vi "Arreglos.vi"() -> ()   [LabVIEW 2020]
uses:
  868cc0ce-591d-4479-aae9-2e439e702293.vi
  d12f55c6-8a29-46e1-aa33-0beeea72b53e.vi
panel:
  out "array out 2":dbl[](array[numeric])
  out "array out":dbl[](array[numeric])
  out "index of element":i32
  out "min index(es)":i32
  out "min value":dbl
  out "max index(es)":i32
  out "max value":dbl
  out "appended array":dbl[](array[numeric])
  in  "Gauge":dbl(knob) scale=0.0..10.0
  in  "Dial":dbl(knob) scale=0.0..10.0
  in  "Knob":dbl(knob) scale=0.0..10.0
  in  "Thermometer":dbl(slide) scale=0.0..100.0
  out "initialized array 2":bool[](array[boolean])
  out "initialized array":dbl[](array[numeric])
  out "subarray":u8[](array[numeric])
  out "output array 2":u8[](array[numeric])
  in  "Nivel Tanque":u8(slide) scale=0.0..10.0
  in  "Velocimetro":u8(knob) scale=0.0..10.0
  out "size(s)":i32
  in  "Array 4":u8[](array[numeric])
  out "element 4":string
  in  "Array 3":string[](array[string])
  out "output array":bool[](array[boolean])
  in  "Array 2":bool[](array[boolean])
  out "element 3":dbl
  out "element 2":dbl
  out "element":dbl
  in  "Array":dbl[](array[slide]) scale=0.0..100.0
  # "Arreglos"
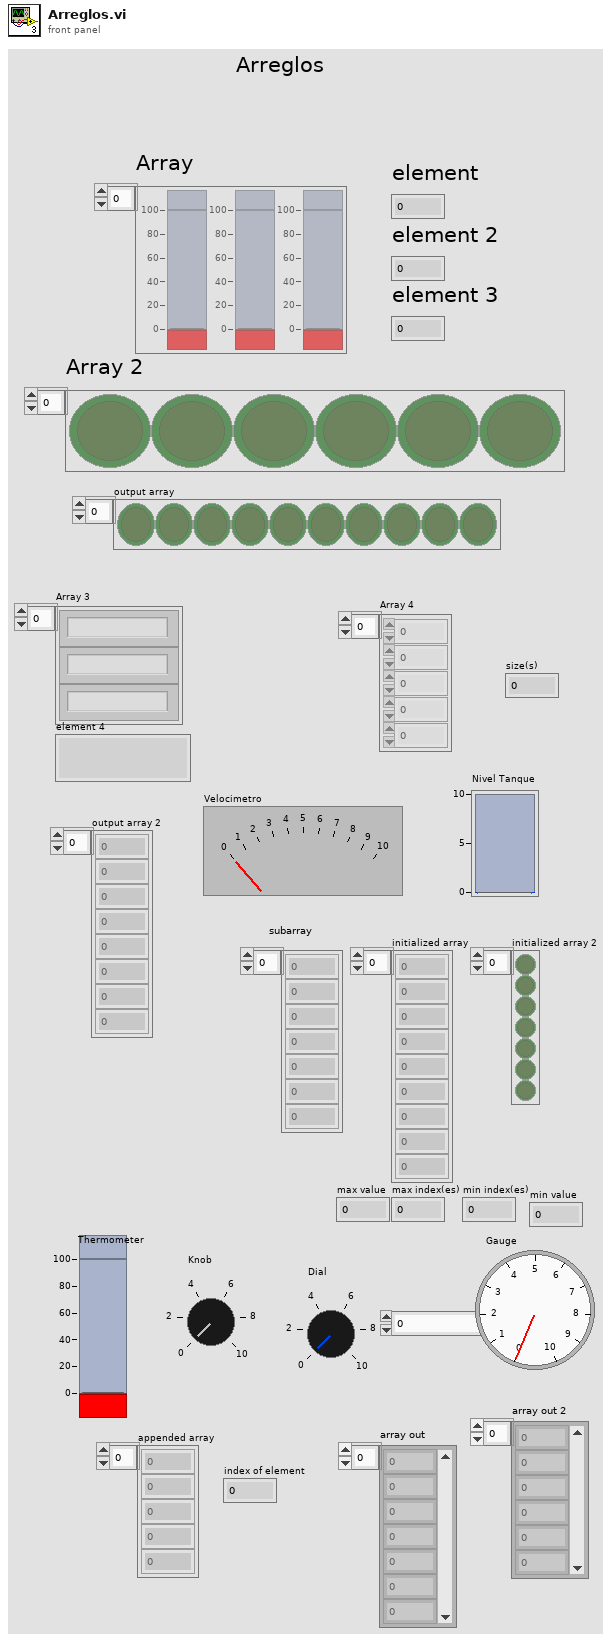
[diagram p1: front panel]
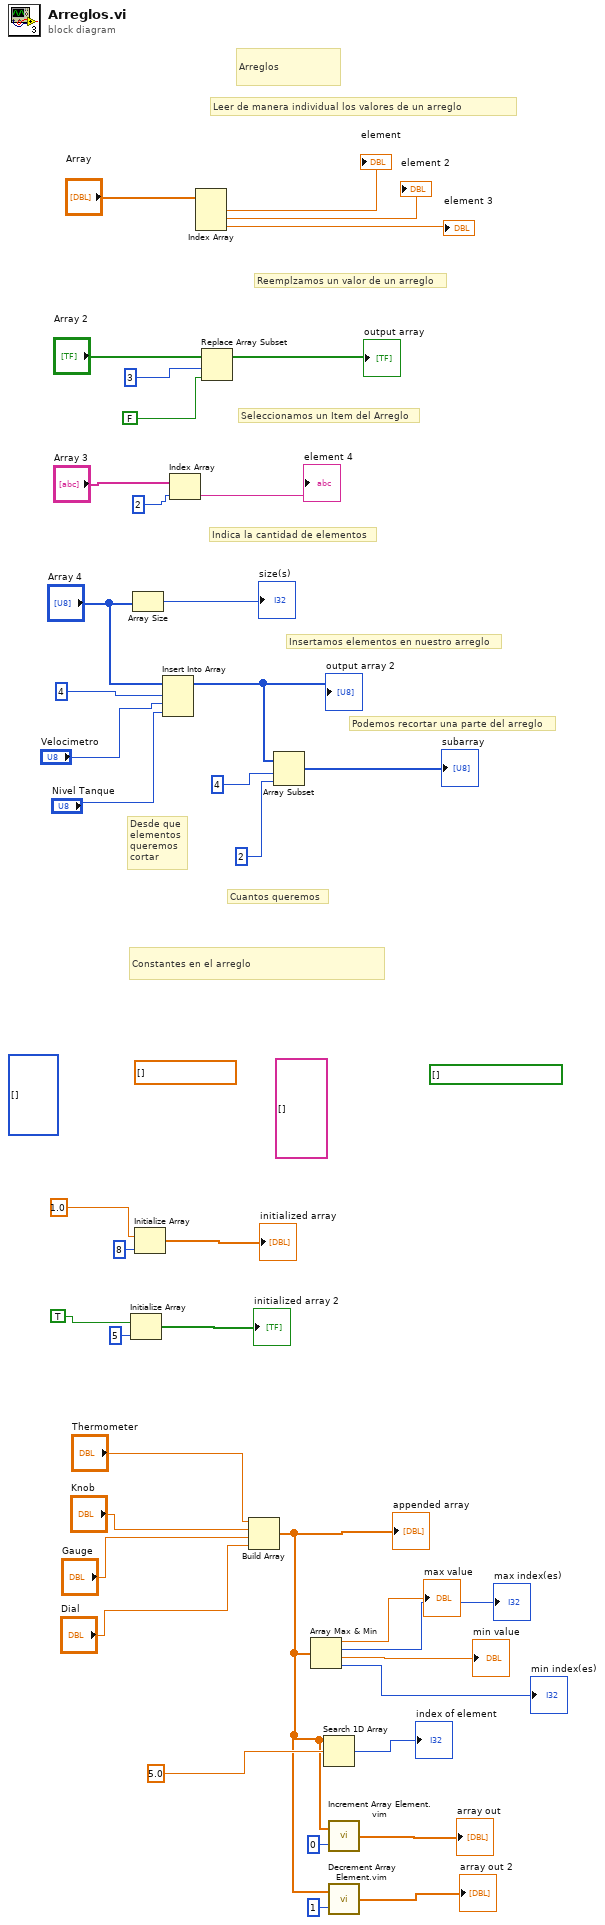
[diagram p0: block diagram]
diagram:
  (unwired) bool[] []
  (unwired) string[] []
  (unwired) dbl[] []
  (unwired) i32[] []
  # "Constantes en el arreglo"
  # "Podemos recortar una parte del arreglo"
  # "Cuantos queremos"
  # "Desde que\nelementos \nqueremos\ncortar"
  # "Insertamos elementos en nuestro arreglo"
  # "Indica la cantidad de elementos"
  # "Seleccionamos un Item del Arreglo"
  # "Reemplzamos un valor de un arreglo"
  # "Leer de manera individual los valores de un arreglo"
  # "Arreglos"
  n1 = Initialize Array(TRUE, 5 ("dimension size")) -> (→"initialized array 2":bool[])
  n2 = Array Size(array="Array 4") -> (size(s)=→"size(s)":i32)
  n3 = Initialize Array(1.0, 8 ("dimension size")) -> (→"initialized array":dbl[])
  n4 = Insert Into Array(array="Array 4", index=4, new element #1="Velocimetro", new element #2="Nivel Tanque") -> (w25:u8[])
  "output array 2" <- w25
  n5 = Index Array(array="Array 3", index=2) -> (element=→"element 4":string)
  n6 = Index Array(array="Array") -> (element #1=→"element":dbl, element #2=→"element 2":dbl, element #3=→"element 3":dbl)  [unwired: 3 in]
  n7 = Replace Array Subset(array="Array 2", new element=FALSE, index=3) -> (→"output array":bool[])
  n8 = Build Array("Thermometer", "Knob", "Gauge", "Dial") -> (w5:dbl[])
  "appended array" <- w5
  n9 = Array Subset(array=w25, index=4, length=2) -> (→"subarray":u8[])
  n10 = Array Max & Min(array=w5) -> (max value=→"max value":dbl, max index (indices)=→"max index(es)":i32, min value=→"min value":dbl, min index (indices)=→"min index(es)":i32)
  n11 = Search 1D Array(1D array=w5, element=5.0) -> (index of element=→"index of element":i32)  [unwired: 1 in]
  n12 = call "Increment Array Element.vim"("index"=0, "array in"=w5) -> ("array out"=→"array out":dbl[])
  n13 = call "Decrement Array Element.vim"("index"=1, "array in"=w5) -> ("array out"=→"array out 2":dbl[])
